vi "Broadcast H2 Sensor Data.vi"(8 "error in":errorcluster, 10 "Data Map":map{string, dbl}(c390)) -> (0 "error out":errorcluster)   [LabVIEW 2024, in "Anode.lvlib"]
doc: "Broadcasts H2 Sensor Data.\n\n_____\nCreated using DQMH Framework: Event Scripter 7.1.1.1528."
uses:
  Anode.lvlib
  Broadcast H2 Sensor Data Argument--cluster.ctl
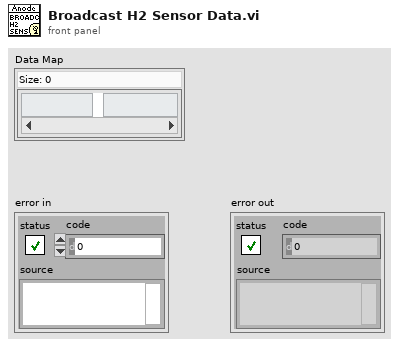
[diagram p1: front panel]
types:
  T1 = typedef "Anode.lvlib/Broadcast H2 Sensor Data Argument--cluster.ctl" = cluster{"Data Map":map{string, dbl}}
  T2 = typedef "Anode.lvlib/Broadcast Events--cluster.ctl" = cluster{"Module Did Init":refnum<user-event>, "Status Updated":refnum<user-event>, "Error Reported":refnum<user-event>, "Module Did Stop":refnum<user-event>, "Update Module Execution Status":refnum<user-event>, "Broadcast Anode State":refnum<user-event>, "Broadcast H2 Sensor Data":refnum<user-event>}
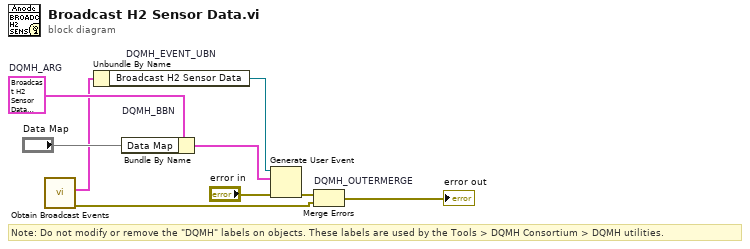
[diagram p0: block diagram]
diagram:
  w4 = T1 {"Data Map"={}}  # DQMH_ARG
  # "Note: Do not modify or remove the \"DQMH\" labels on objects. These labels are used by the Tools > DQMH Consortium > DQMH utilities."
  n1 = call "Obtain Broadcast Events.vi"() -> ("error out"=w2:errorcluster, "Anode Broadcast Events"=w1:T2)  [unwired: 10 in]
  n2 = Unbundle By Name "DQMH_EVENT_UBN"(w1) -> ("Broadcast H2 Sensor Data"=w6:refnum<user-event>)
  n3 = Bundle By Name "DQMH_BBN"(cluster=w4, "Data Map"="Data Map") -> (w7:T1)
  n4 = Generate User Event(user event=w6, event data cluster=w7, error in="error in") -> (error out=w5:errorcluster)  [unwired: 1 in, 1 out]
  n5 = Merge Errors "DQMH_OUTERMERGE"(w5, w2) -> (→"error out":errorcluster)
